vi "Read Waveform.vi"(8 "error in (no error)":errorcluster, 11 "Agilent DSO1000 in":refnum<class "Agilent DSO1000.lvclass">) -> (0 "error out":errorcluster, 2 "Waveform Data":waveform(dbl)[](graph), 3 "Agilent DSO1000 out":refnum<class "Agilent DSO1000.lvclass">)   [LabVIEW 2020, in "Agilent DSO1000.lvclass"]
uses:
  Agilent DSO1000.lvclass
  C:/Sandbox/Git_Sandbox/WiSpry Test Framework source code (LV20)/WiSpry Test Framework/Instruments/Instrument.lvclass
  Instrument.lvclass/Instrument.ctl
  <instrlib>/Agilent DSO1000 Series/Public/Data/Read Waveform (Multiple).vi
  Instrument.lvclass
  <instrlib>/Agilent DSO1000 Series/Agilent DSO1000 Series.lvlib
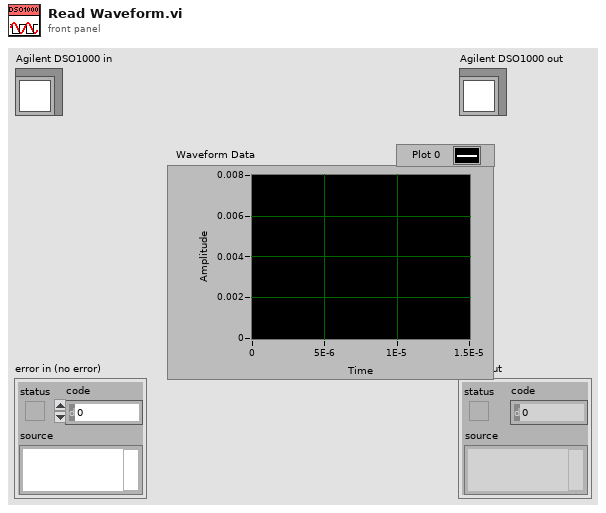
[diagram p1: front panel]
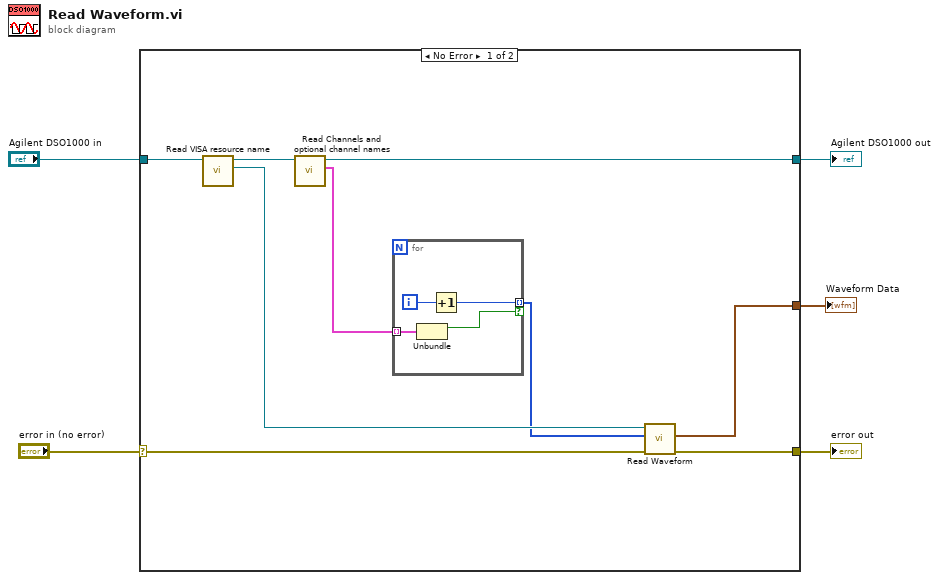
[diagram p0: block diagram]
diagram:
  n1 = case shown="No Error" "error in (no error)" {
    selector: "error in (no error)" -> [w12 w20]
    tunnel: [w7 w20] -> w4
    tunnel: [w10 w19] -> w3
    tunnel: "Agilent DSO1000 in" -> [w14 w19]
    tunnel: [w6 _] -> w1
    frame No Error {
      n2 = call "Read VISA resource name.vi"("Instrument in"=w14) -> ("VISA resource name"=w11:refnum<visa-resource-name>, "Instrument out"=w13:refnum<class "Agilent DSO1000.lvclass">)  [unwired: 9 in]
      n3 = call-dynamic "Read Channels and optional channel names.vi"("Oscilloscope in"=w13) -> ("Channels and optional channel names"=w9:cluster{"Enabled":bool, "Channel name":string}[], "Oscilloscope out"=w10:refnum<class "Agilent DSO1000.lvclass">)  [unwired: 9 in]
      n4 = for {
        tunnel: w9 -> [w18] mode=indexing
        tunnel: [w16] -> w8 mode=indexing if=w15
        i -> [w17]
        n5 = Unbundle(w18) -> ("Enabled"=w15:bool)  [unwired: 1 out]
        n6 = Increment(x=w17) -> (x+1=w16:i32)
      }
      n7 = call-poly <instrlib>:"Read Waveform.vi"("error in (no error)"=w12, "Channels"=w8, "VISA resource name"=w11) -> ("error out"=w7:errorcluster, "Waveform Data"=w6:waveform(dbl)[])  [unwired: 6 in, 1 out]
    }
    frame Error {
    }
  }
  "error out" <- w4
  "Agilent DSO1000 out" <- w3
  "Waveform Data" <- w1
